vi "Create-reference.vi"(8 "error in (no error)":errorcluster) -> (0 "error out":errorcluster, 3 "Data ref.":refnum<data-value>)   [LabVIEW 2013, in "CameraVision.lvlib" / "CV-Main.lvclass"]
uses:
  CV-Main.lvclass
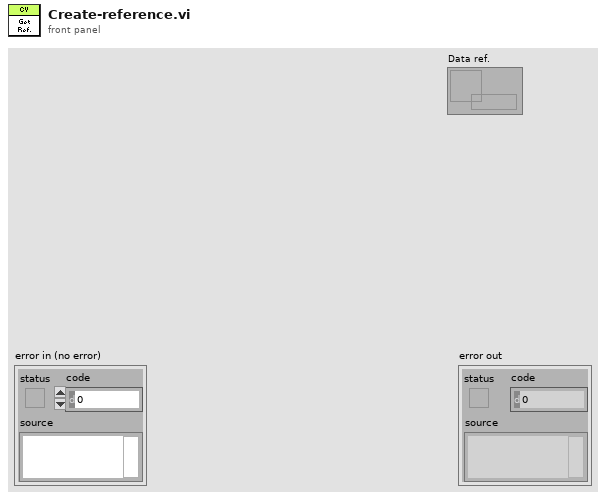
[diagram p1: front panel]
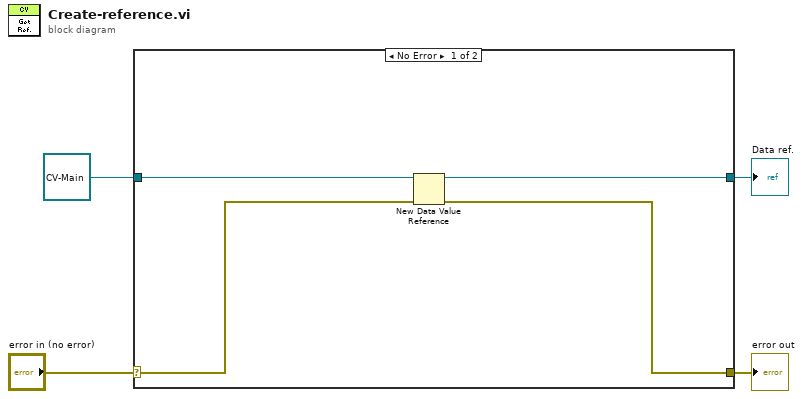
[diagram p0: block diagram]
diagram:
  n1 = case shown="No Error" "error in (no error)" {
    selector: "error in (no error)" -> [w5 w9]
    tunnel: [w8 w9] -> w3
    tunnel: refnum<class "CV-Main.lvclass"> refnum ("Data in") -> [w6 _]
    tunnel: [w7 _] -> w1
    frame No Error {
      n2 = New Data Value Reference(data value=w6, error in=w5) -> (data value reference=w7:refnum<data-value>, error out=w8:errorcluster)
    }
    frame Error {
    }
  }
  "error out" <- w3
  "Data ref." <- w1
